vi "Get Data.vi"(8 "error in":errorcluster, 11 "nPAS in":refnum<class "nPAS.lvclass">) -> (0 "error out":errorcluster, 3 "nPAS out":refnum<class "nPAS.lvclass">)   [LabVIEW 2015, in "nPAS.lvclass"]
doc: "Here you will do all of your acquisition. The acquisition is going to be implementation dependent, but at the bare minimum the class which inherits the PAS will have to retrieve the speaker signal(s). The data that is acquired in this cycle will be piped to the <b>Analyze Data</b> VI in the next cycle."
uses:
  nPAS.lvclass
  Session/Raw FPGA/FPGA Session.lvclass
  nPAS.lvclass/nPAS.ctl
  Session/Raw FPGA/FPGA Session.lvclass/FPGA Session.ctl
  Session/Raw FPGA/Read FPGA Ref.vi
  <vilib>/Utility/error.llb/Error Cluster From Error Code.vi
  <vilib>/rvi/errors/niLvFpgaAdjustHostInterfaceError.vi
  FPGA Ref.ctl
  <vilib>/rvi/interface/nirviMethod/nirviMethod.xnode
  FPGA Bitfiles/NickIO.lvbitx
  Reusable/PAS/Main/PAS.lvclass
  Reusable/PAS/Data/Cell/PAS Cell Data.lvclass
  Reusable/Data/Data.lvclass
  <vilib>/FPGAPlugInAG/cRIO-9081/niLvFpga_ReadFifo_cRIO-9081.vi
  <vilib>/rvi/errors/niLvFpgaMergeErrorWithErrorCode.vi
panel:
  out "Elements Remaining":u32
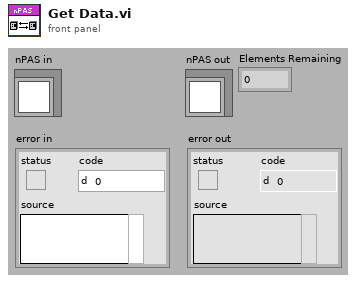
[diagram p1: front panel]
types:
  T1 = typedef "Session - Root.lvclass/Session Handle.ctl" = refnum<data-value>
  T2 = typedef "FPGA Ref.ctl" = refnum<k20>
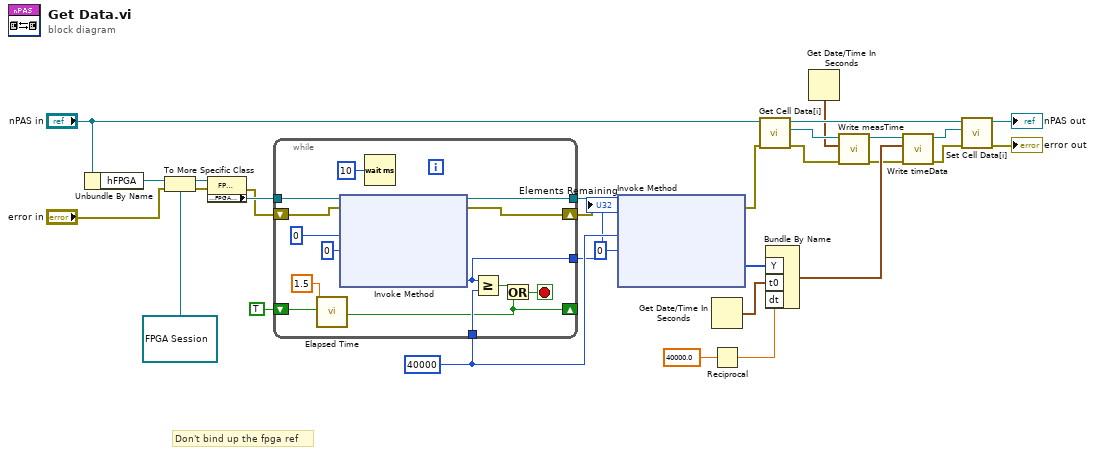
[diagram p0: block diagram]
diagram:
  w3 = u32 40000 ("Number of Elements")
  # "Don't bind up the fpga ref"
  n1 = Unbundle By Name("nPAS in") -> ("hFPGA"=w20:T1)
  n2 = To More Specific Class(target class=refnum<data-value> refnum ("hFPGA"), reference=w20, error in="error in") -> (specific class reference=w17:refnum<data-value>, error out=w16:errorcluster)
  n3 = property class="FPGA Session"(reference=w17, error in=w16) -> (error out=w14:errorcluster, "Accessors:FPGA Ref"=w15:T2)  [unwired: 1 out]
  n4 = while {
    tunnel: w15 -> [w43]
    shift-right: [w44] -> w7
    shift-left: w14 -> [w42]
    tunnel: [w39] -> w8
    shift-right: [w35] -> _
    shift-left: TRUE ("Time has Elapsed") -> [w38]
    tunnel: w3 -> [w37]
    tunnel: [w32] -> w1
    stop <- w34 stop-if-true
    n5 = call "Elapsed Time"("Time Target (s)"=1.5 ("Set Start Time (s)"), "Reset"=w38) -> ("Time has Elapsed"=w35:bool)  [unwired: 10 in, 7 out]
    n6 = xnode "Invoke Method"("FPGA VI Reference In"=w43, "error in"=w42, "Number of Elements"=u32 0, "Timeout (ms)"=0) -> ("FPGA VI Reference Out"=w39:T2, "error out"=w44:errorcluster, "Elements Remaining"=w32:u32)  [unwired: 1 out]
    n7 = Wait (ms)(milliseconds to wait=u32 10) -> ()  [unwired: 1 out]
    n8 = Greater Or Equal?(x=w32, y=w37) -> (x >= y?=w36:bool)
    n9 = Or(x=w36, y=w35) -> (x .or. y?=w34:bool)
  }
  "Elements Remaining" <- w1
  n10 = xnode "Invoke Method"("FPGA VI Reference In"=w8, "error in"=w7, "Number of Elements"=w3, "Timeout (ms)"=0) -> ("error out"=w5:errorcluster, "Data"=w2:i16[])  [unwired: 2 out]
  n11 = Get Date/Time In Seconds() -> (seconds since 1Jan1904=w29:timestamp)
  n12 = Reciprocal(x=40000.0) -> (1/x=w27:dbl)
  n13 = call "Get Cell Data[i].vi"("error in (no error)"=w5, "PAS in"="nPAS in") -> ("error out"=w11:errorcluster, "Cell Data[i]"=w13:refnum<class "PAS Cell Data.lvclass">, "PAS out"=w24:refnum<class "nPAS.lvclass">)  [unwired: 7 in]
  n14 = Bundle By Name("Y"=w2, "t0"=w29, "dt"=w27) -> (w26:waveform(i16))  [unwired: 1 in]
  n15 = Get Date/Time In Seconds() -> (seconds since 1Jan1904=w9:timestamp)
  n16 = call "Write measTime.vi"("error in (no error)"=w11, "measTime"=w9, "Data in"=w13) -> ("error out"=w10:errorcluster, "Data out"=w12:refnum<class "PAS Cell Data.lvclass">)  [unwired: 7 in]
  n17 = call "Write timeData.vi"("error in (no error)"=w10, "timeData"=w26, "PAS Cell Data in"=w12) -> ("error out"=w23:errorcluster, "PAS Cell Data out"=w25:refnum<class "PAS Cell Data.lvclass">)  [unwired: 7 in]
  n18 = call "Set Cell Data[i].vi"("error in (no error)"=w23, "Cell Data[i]"=w25, "PAS in"=w24) -> ("error out"=→"error out":errorcluster, "PAS out"=→"nPAS out":refnum<class "nPAS.lvclass">)  [unwired: 7 in]
